vi "gVar_ECa2.vi"() -> ()   [LabVIEW 2020]
panel:
  out "ECa2":dbl
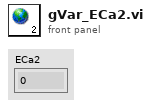
[diagram p1: front panel]
diagram:
